vi "Translator ID Nums.vi"(10 "Driver Label":T3, 11 "Manipulator Label":T4) -> (2 "Driver Control Indexes":T1, 3 "Manipulator Control Indexes":T2)   [LabVIEW 2015]
uses:
  Common Code/Manipulator Control Label.ctl
  Common Code/Driver Control Label.ctl
  Common Code/Manipulator Control Indexes.ctl
  Common Code/Driver Control Indexes.ctl
panel:
  out "Array":i32[](array[numeric])
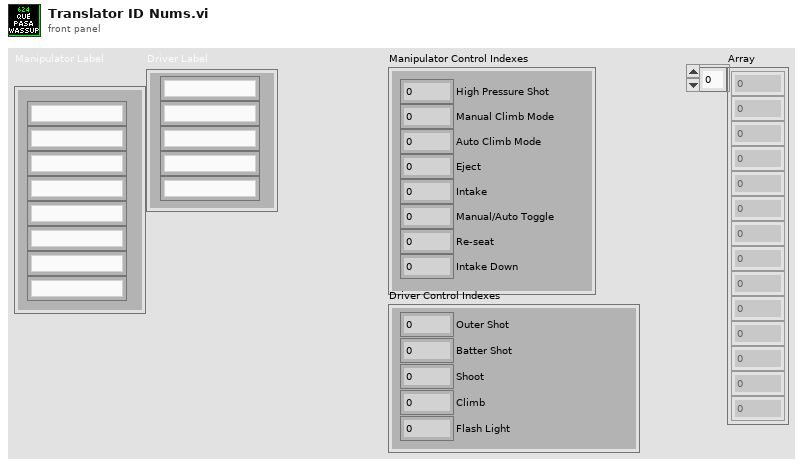
[diagram p1: front panel]
types:
  T1 = typedef "Driver Control Indexes.ctl" = cluster{"Outer Shot":dbl, "Batter Shot":dbl, "Shoot":dbl, "Climb":dbl, "Flash Light":dbl}
  T2 = typedef "Manipulator Control Indexes.ctl" = cluster{"High Pressure Shot":dbl, "Manual Climb Mode":dbl, "Auto Climb Mode":dbl, "Eject":dbl, "Intake":dbl, "Manual/Auto Toggle":dbl, "Re-seat":dbl, "Intake Down":dbl}
  T3 = typedef "Driver Control Label.ctl" = cluster{"Outer Shot":string, "Batter Shot":string, "Shoot":string, "Climb":string, "Flashlight":string}
  T4 = typedef "Manipulator Control Label.ctl" = cluster{"High Pressure Shot":string, "Manual Climb Mode":string, "Auto Climb Mode":string, "Eject":string, "Intake":string, "Manual/Auto Toggle":string, "Re-seat":string, "Intake Down":string}
  T5 = cluster{"[0]":i32, "[1]":i32, "[2]":i32, "[3]":i32, "[4]":i32, "[5]":i32, "[6]":i32, "[7]":i32}
  T6 = cluster{"[0]":i32, "[1]":i32, "[2]":i32, "[3]":i32, "[4]":i32}
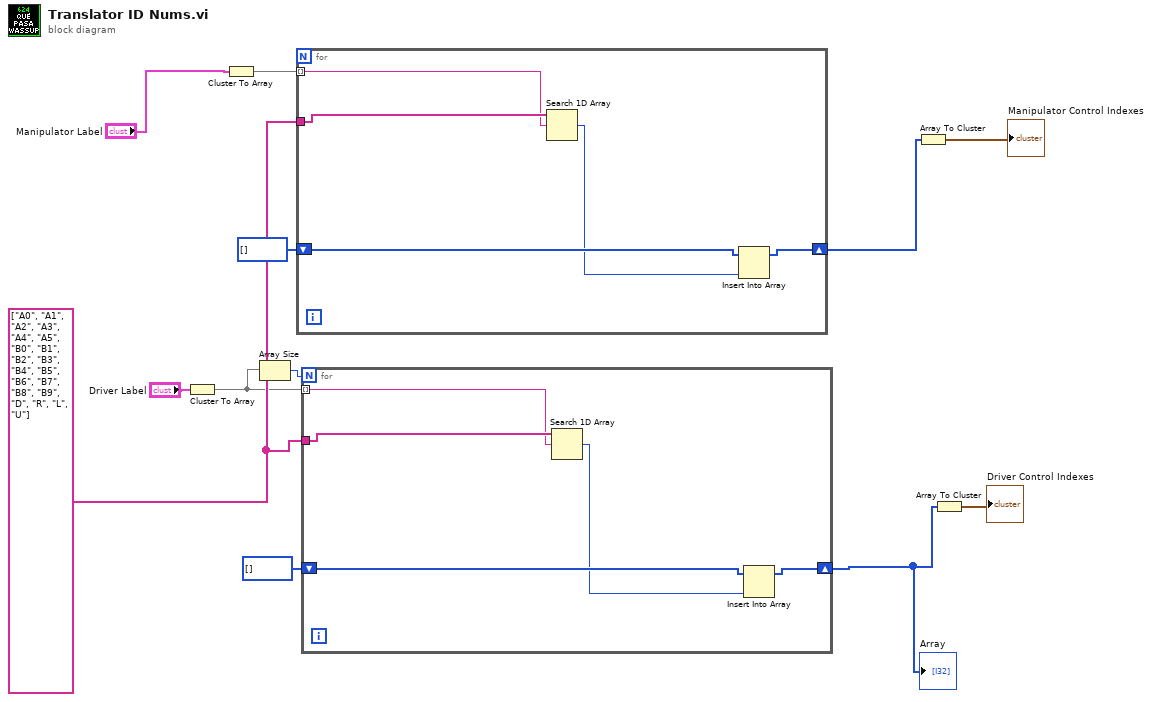
[diagram p0: block diagram]
diagram:
  w10 = string[] ["A0", "A1", "A2", "A3", "A4", "A5", "B0", "B1", "B2", "B3", "B4", "B5", "B6", "B7", "B8", "B9", "D", "R", "L", "U"]
  n1 = Cluster To Array(cluster="Driver Label") -> (array=w6:string[])
  n2 = Cluster To Array(cluster="Manipulator Label") -> (array=w8:string[])
  n3 = Array Size(array=w6) -> (size(s)=w7:i32)
  n4 = for {
    tunnel: w10 -> [w17]
    shift-right: [w16] -> w2
    shift-left: i32[] [] -> [w15]
    tunnel: w8 -> [w13] mode=indexing
    n5 = Search 1D Array(1D array=w17, element=w13) -> (index of element=w14:i32)  [unwired: 1 in]
    n6 = Insert Into Array(array=w15, new element=w14) -> (w16:i32[])  [unwired: 1 in]
  }
  n7 = for {
    N: w7 -> [_]
    tunnel: w6 -> [w21] mode=indexing
    tunnel: w10 -> [w22]
    shift-right: [w20] -> w11
    shift-left: i32[] [] -> [w19]
    n8 = Search 1D Array(1D array=w22, element=w21) -> (index of element=w18:i32)  [unwired: 1 in]
    n9 = Insert Into Array(array=w19, new element=w18) -> (w20:i32[])  [unwired: 1 in]
  }
  "Array" <- w11
  n10 = Array To Cluster(array=w2) -> (cluster=→"Manipulator Control Indexes":T5)
  n11 = Array To Cluster(array=w11) -> (cluster=→"Driver Control Indexes":T6)
